vi "Set Number.vi"(6 "timeout (ms)":i32=5000, 8 "error in":errorcluster, 10 "SetNumber":u32, 11 "gRPC ID":T1) -> (0 "error out":errorcluster, 3 "gRPC ID out":T1)   [LabVIEW 2023, in "AMSCyclerTemplateService_Client_Wrapper.lvlib"]
uses:
  AMSCyclerTemplateService_Client_Wrapper.lvlib
  <vilib>/gRPC/LabVIEW gRPC Library/Shared/grpcId.ctl
  AMSCyclerTemplateService_client/RPC Messages/adas_SetNumberRequest.ctl
  AMSCyclerTemplateService_client/AMSCyclerTemplateService_client.lvlib
  <vilib>/gRPC/LabVIEW gRPC Library/grpc-lvsupport-release.lvlib
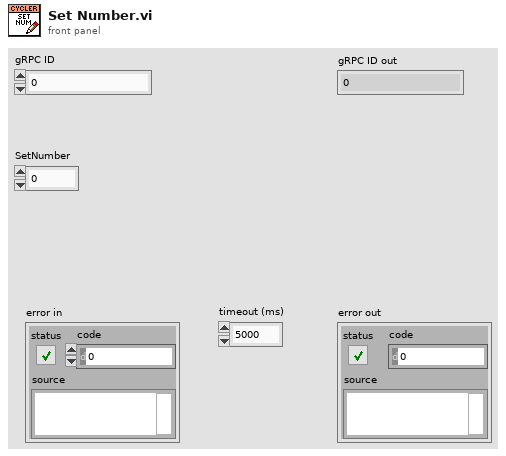
[diagram p1: front panel]
types:
  T1 = typedef "grpc-lvsupport-release.lvlib/grpcId.ctl" = u64
  T2 = typedef "AMSCyclerTemplateService_client.lvlib/adas_SetNumberRequest.ctl" = cluster{"SetNumber":u32}
  T3 = typedef "AMSCyclerTemplateService_client.lvlib/adas_Status.ctl" = cluster{"Code":i32, "Message":string}
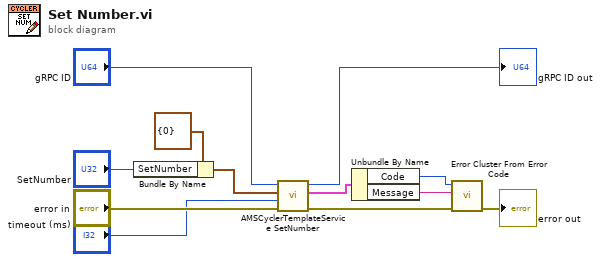
[diagram p0: block diagram]
diagram:
  n1 = Bundle By Name(cluster=T2 {"SetNumber"=0} ("Request Data"), "SetNumber"="SetNumber") -> (w8:T2)
  n2 = call "AMSCyclerTemplateService SetNumber.vi"("error in"="error in", "timeout (ms)"="timeout (ms)", "Request Data"=w8, "gRPC ID"="gRPC ID") -> ("error out"=w2:errorcluster, "Response Data"=w3:T3, "gRPC ID out"=→"gRPC ID out":T1)  [unwired: 5 in]
  n3 = Unbundle By Name(w3) -> ("Code"=w4:i32, "Message"=w5:string)
  n4 = call <vilib>:"Error Cluster From Error Code.vi"("error in (no error)"=w2, "error message (\"\")"=w5, "error code (0)"=w4) -> ("error out"=→"error out":errorcluster)  [unwired: 6 in]
